vi "Buttons.vi"() -> ()   [LabVIEW 2012]
uses:
  GUI_Buttons_23x22_W2K.llb/JumpNext.ctl
  GUI_Buttons_23x22_W2K.llb/SearchFiles.ctl
  GUI_Buttons_23x22_W2K.llb/Search.ctl
  GUI_Buttons_23x22_W2K.llb/Paste.ctl
  GUI_Buttons_23x22_W2K.llb/Wrap.ctl
  GUI_Buttons_23x22_W2K.llb/Undo.ctl
  GUI_Buttons_23x22_W2K.llb/New.ctl
  GUI_Buttons_23x22_W2K.llb/Open.ctl
  GUI_Buttons_23x22_W2K.llb/Save.ctl
  GUI_Buttons_23x22_W2K.llb/Print.ctl
  GUI_Buttons_23x22_W2K.llb/Preview.ctl
  GUI_Buttons_23x22_W2K.llb/MacroRecord.ctl
  GUI_Buttons_23x22_W2K.llb/MacroPause.ctl
  GUI_Buttons_23x22_W2K.llb/MacroStop.ctl
  GUI_Buttons_23x22_W2K.llb/MacroPlay.ctl
  GUI_Buttons_23x22_W2K.llb/Replace.ctl
  GUI_Buttons_23x22_W2K.llb/Help.ctl
  GUI_Buttons_23x22_W2K.llb/HelpCursor.ctl
  GUI_Buttons_23x22_W2K.llb/JumpPrevious.ctl
  GUI_Buttons_23x22_W2K.llb/HelpBubble.ctl
  GUI_Buttons_23x22_W2K.llb/Cut.ctl
  GUI_Buttons_23x22_W2K.llb/Copy.ctl
  GUI_Buttons_23x22_W2K.llb/Cabinet.ctl
  GUI_Buttons_23x22_W2K.llb/Bullets.ctl
  GUI_Buttons_23x22_W2K.llb/EditDoc.ctl
  GUI_Buttons_23x22_W2K.llb/BarGraph.ctl
  GUI_Buttons_23x22_W2K.llb/Attach.ctl
  GUI_Buttons_23x22_W2K.llb/FileGroup_1.ctl
  GUI_Buttons_23x22_W2K.llb/PrintGroup_1.ctl
  GUI_Buttons_23x22_W2K.llb/EditGroup_1.ctl
  GUI_Buttons_23x22_W2K.llb/EditGroup_2.ctl
  GUI_Buttons_23x22_W2K.llb/MacroGroup_2.ctl
  GUI_Buttons_23x22_W2K.llb/MacroGroup_1.ctl
  GUI_Buttons_23x22_W2K.llb/FileGroup_2.ctl
  GUI_Buttons_23x22_W2K.llb/FindGroup_1.ctl
  GUI_Buttons_23x22_W2K.llb/HelpGroup_1.ctl
  GUI_Buttons_23x22_W2K.llb/HelpGroup_2.ctl
  GUI_Buttons_23x22_W2K.llb/HelpGroup_3.ctl
  GUI_Buttons_23x22_W2K.llb/Link.ctl
  GUI_Buttons_23x22_W2K.llb/LinkBreak.ctl
  GUI_Buttons_23x22_W2K.llb/LinksGroup_1.ctl
  GUI_Buttons_23x22_W2K.llb/ExpandAll.ctl
  GUI_Buttons_23x22_W2K.llb/Expand.ctl
  GUI_Buttons_23x22_W2K.llb/Contract.ctl
  GUI_Buttons_23x22_W2K.llb/Users.ctl
  GUI_Buttons_23x22_W2K.llb/Notes1.ctl
  GUI_Buttons_23x22_W2K.llb/FilterEquals.ctl
  GUI_Buttons_23x22_W2K.llb/Email1.ctl
  GUI_Buttons_23x22_W2K.llb/ArrowLeftBlue.ctl
  GUI_Buttons_23x22_W2K.llb/ArrowRightBlue.ctl
  GUI_Buttons_23x22_W2K.llb/ZoomIn.ctl
  GUI_Buttons_23x22_W2K.llb/ZoomOut.ctl
  GUI_Buttons_23x22_W2K.llb/Camera1.ctl
  GUI_Buttons_23x22_W2K.llb/Wizard.ctl
  GUI_Buttons_23x22_W2K.llb/WizardColors.ctl
  GUI_Buttons_23x22_W2K.llb/Function1.ctl
  GUI_Buttons_23x22_W2K.llb/ClipboardClear.ctl
  GUI_Buttons_23x22_W2K.llb/PropertyFormat1.ctl
  GUI_Buttons_23x22_W2K.llb/IndexCard1.ctl
  GUI_Buttons_23x22_W2K.llb/MoveToFolder.ctl
  GUI_Buttons_23x22_W2K.llb/Delete1.ctl
  GUI_Buttons_23x22_W2K.llb/Book1.ctl
  GUI_Buttons_23x22_W2K.llb/AlphaSortAscending.ctl
  GUI_Buttons_23x22_W2K.llb/Summation.ctl
  GUI_Buttons_23x22_W2K.llb/Hyperlink1.ctl
  GUI_Buttons_23x22_W2K.llb/Table1.ctl
  GUI_Buttons_23x22_W2K.llb/ByRow.ctl
  GUI_Buttons_23x22_W2K.llb/ByCol.ctl
  GUI_Buttons_23x22_W2K.llb/Controls1.ctl
  GUI_Buttons_23x22_W2K.llb/Image1.ctl
  GUI_Buttons_23x22_W2K.llb/ViewText1.ctl
  GUI_Buttons_23x22_W2K.llb/DesignMode1.ctl
panel:
  in  "DesignMode1":T1
  in  "ViewText":T2
  in  "Image1":T3
  in  "Controls1-Up":T4
  in  "ByCol":T5
  in  "ByRow":T6
  in  "Table1":T7
  in  "HyperLink1":T8
  in  "Summation":T9
  in  "AlphaSortAscending":T10
  in  "Book1":T11
  in  "Delete1":T12
  in  "MoveToFolder":T13
  in  "IndexCard1":T14
  in  "PropertyFormat1":T15
  in  "ClipboardClear":T16
  in  "Function1":T17
  in  "WizardColors":T18
  in  "Wizard":T19
  in  "Camera1":T20
  in  "ZoomOut":T21
  in  "ZoomIn":T22
  in  "ArrowRightBlue":T23
  in  "ArrowLeftBlue":T24
  in  "Email1":T25
  in  "FilterEquals":T26
  in  "Notes1":T27
  in  "Users":T28
  in  "Contract":T29
  in  "Expand":T30
  in  "ExpandAll":T31
  in  "LinksGroup_1":T32
  in  "LinkBreak":T34
  in  "Link":T33
  in  "Boolean":bool
  in  "HelpGroup_3":T35
  in  "HelpGroup_2":T38
  in  "HelpGroup_1":T40
  in  "FindGroup_1":T41
  in  "FileGroup_2":T45
  in  "MacroGroup_1":T50
  in  "MacroGroup_2":T55
  in  "EditGroup_2":T56
  in  "EditGroup_1":T61
  in  "PrintGroup_1":T62
  in  "Cluster":cluster{}
  in  "FileGroup_1":T65
  in  "Attach":T66
  in  "BarGraph":T67
  in  "EditDoc":T68
  in  "Bullets":T69
  in  "Cabinet":T49
  in  "HelpBubble":T37
  in  "JumpPrevious":T70
  in  "HelpCursor":T36
  in  "Help":T39
  in  "Replace":T44
  in  "MacroPlay":T51
  in  "MacroStop":T53
  in  "MacroPause":T52
  in  "MacroRecord":T54
  in  "JumpNext":T71
  in  "SearchFiles":T43
  in  "Search":T42
  in  "Undo":T60
  in  "Wrap":T72
  in  "Preview":T64
  in  "Print":T63
  in  "Save":T48
  in  "Open":T47
  in  "New":T46
  in  "Paste":T59
  in  "Copy":T58
  in  "Cut":T57
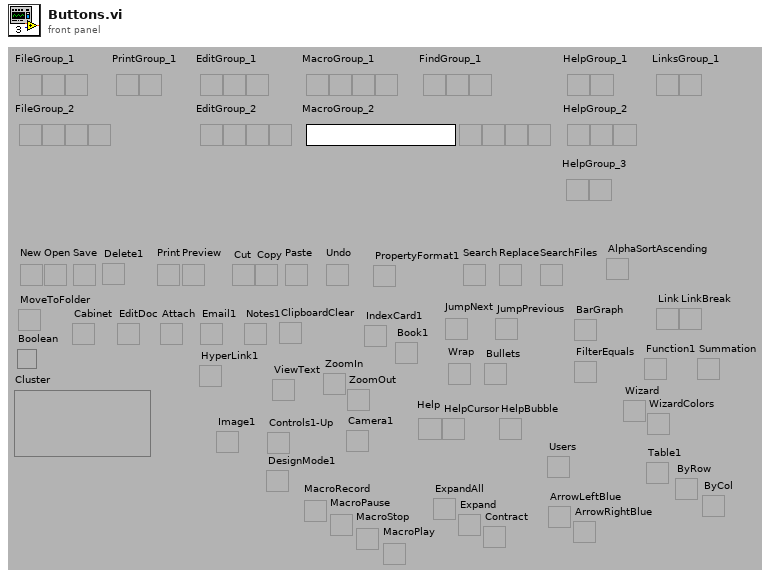
[diagram p1: front panel]
types:
  T1 = typedef "DesignMode1.ctl" = bool
  T2 = typedef "ViewText1.ctl" = bool
  T3 = typedef "Image1.ctl" = bool
  T4 = typedef "Controls1.ctl" = bool
  T5 = typedef "ByCol.ctl" = bool
  T6 = typedef "ByRow.ctl" = bool
  T7 = typedef "Table1.ctl" = bool
  T8 = typedef "Hyperlink1.ctl" = bool
  T9 = typedef "Summation.ctl" = bool
  T10 = typedef "AlphaSortAscending.ctl" = bool
  T11 = typedef "Book1.ctl" = bool
  T12 = typedef "Delete1.ctl" = bool
  T13 = typedef "MoveToFolder.ctl" = bool
  T14 = typedef "IndexCard1.ctl" = bool
  T15 = typedef "PropertyFormat1.ctl" = bool
  T16 = typedef "ClipboardClear.ctl" = bool
  T17 = typedef "Function1.ctl" = bool
  T18 = typedef "WizardColors.ctl" = bool
  T19 = typedef "Wizard.ctl" = bool
  T20 = typedef "Camera1.ctl" = bool
  T21 = typedef "ZoomOut.ctl" = bool
  T22 = typedef "ZoomIn.ctl" = bool
  T23 = typedef "ArrowRightBlue.ctl" = bool
  T24 = typedef "ArrowLeftBlue.ctl" = bool
  T25 = typedef "Email1.ctl" = bool
  T26 = typedef "FilterEquals.ctl" = bool
  T27 = typedef "Notes1.ctl" = bool
  T28 = typedef "Users.ctl" = bool
  T29 = typedef "Contract.ctl" = bool
  T30 = typedef "Expand.ctl" = bool
  T31 = typedef "ExpandAll.ctl" = bool
  T32 = typedef "LinksGroup_1.ctl" = cluster{"Link":T33, "LinkBreak":T34}
  T33 = typedef "Link.ctl" = bool
  T34 = typedef "LinkBreak.ctl" = bool
  T35 = typedef "HelpGroup_3.ctl" = cluster{"HelpCursor":T36, "HelpBubble":T37}
  T36 = typedef "HelpCursor.ctl" = bool
  T37 = typedef "HelpBubble.ctl" = bool
  T38 = typedef "HelpGroup_2.ctl" = cluster{"HelpCursor":T36, "HelpBubble":T37, "Help":T39}
  T39 = typedef "Help.ctl" = bool
  T40 = typedef "HelpGroup_1.ctl" = cluster{"HelpCursor":T36, "Help":T39}
  T41 = typedef "FindGroup_1.ctl" = cluster{"Search":T42, "SearchFiles":T43, "Replace":T44}
  T42 = typedef "Search.ctl" = bool
  T43 = typedef "SearchFiles.ctl" = bool
  T44 = typedef "Replace.ctl" = bool
  T45 = typedef "FileGroup_2.ctl" = cluster{"New":T46, "Open":T47, "Save":T48, "Cabinet":T49}
  T46 = typedef "New.ctl" = bool
  T47 = typedef "Open.ctl" = bool
  T48 = typedef "Save.ctl" = bool
  T49 = typedef "Cabinet.ctl" = bool
  T50 = typedef "MacroGroup_1.ctl" = cluster{"MacroPlay":T51, "MacroPause":T52, "MacroStop":T53, "MacroRecord":T54}
  T51 = typedef "MacroPlay.ctl" = bool
  T52 = typedef "MacroPause.ctl" = bool
  T53 = typedef "MacroStop.ctl" = bool
  T54 = typedef "MacroRecord.ctl" = bool
  T55 = typedef "MacroGroup_2.ctl" = cluster{"MacroPlay":T51, "MacroPause":T52, "MacroStop":T53, "MacroRecord":T54, "MacroName":u16}
  T56 = typedef "EditGroup_2.ctl" = cluster{"Cut":T57, "Copy":T58, "Paste":T59, "Undo":T60}
  T57 = typedef "Cut.ctl" = bool
  T58 = typedef "Copy.ctl" = bool
  T59 = typedef "Paste.ctl" = bool
  T60 = typedef "Undo.ctl" = bool
  T61 = typedef "EditGroup_1.ctl" = cluster{"Cut":T57, "Copy":T58, "Paste":T59}
  T62 = typedef "PrintGroup_1.ctl" = cluster{"Print":T63, "Preview":T64}
  T63 = typedef "Print.ctl" = bool
  T64 = typedef "Preview.ctl" = bool
  T65 = typedef "FileGroup_1.ctl" = cluster{"New":T46, "Open":T47, "Save":T48}
  T66 = typedef "Attach.ctl" = bool
  T67 = typedef "BarGraph.ctl" = bool
  T68 = typedef "EditDoc.ctl" = bool
  T69 = typedef "Bullets.ctl" = bool
  T70 = typedef "JumpPrevious.ctl" = bool
  T71 = typedef "JumpNext.ctl" = bool
  T72 = typedef "Wrap.ctl" = bool
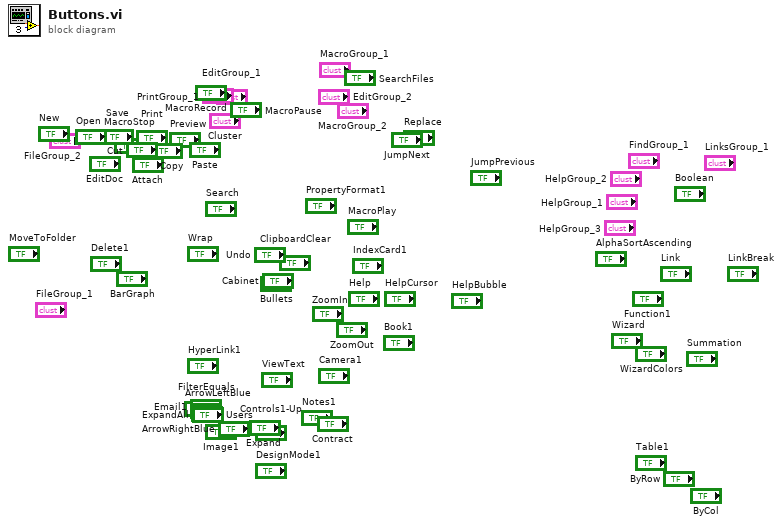
[diagram p0: block diagram]
diagram:
